vi "createXMLNode.vi"(8 "error in (no error)":errorcluster, 11 "name":string) -> (0 "error out":errorcluster, 3 "xmlNode out":refnum<class "xmlNode.lvclass">)   [LabVIEW 2011, in "Tools.lvlib" / "xml.lvlib" / "xmlNode.lvclass"]
uses:
  xmlNode.lvclass
  xmlNode.lvclass/xmlNode.ctl
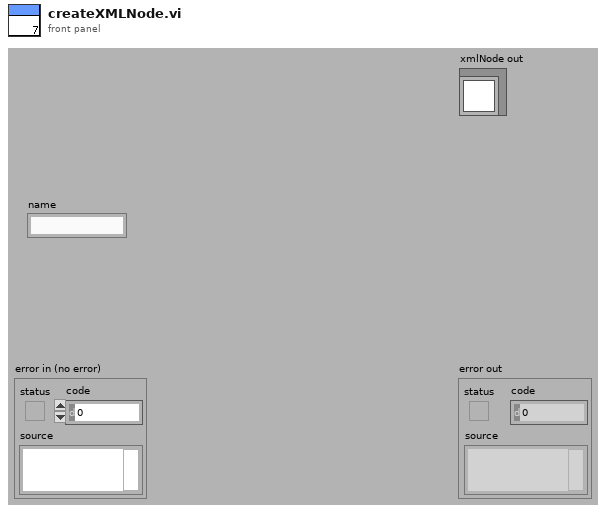
[diagram p1: front panel]
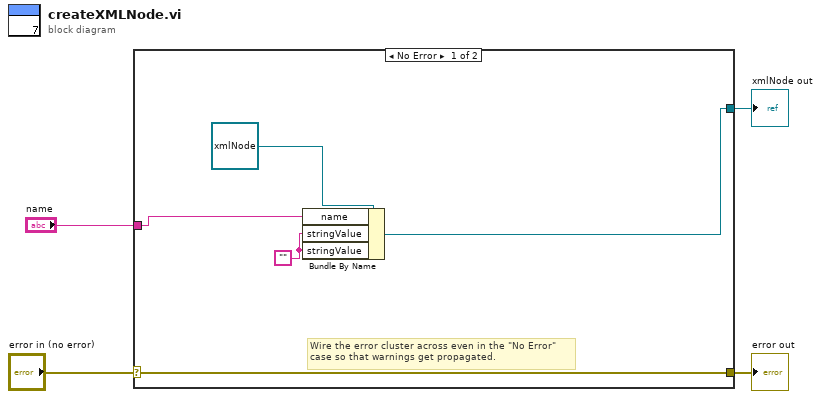
[diagram p0: block diagram]
diagram:
  n1 = case shown="No Error" "error in (no error)" {
    selector: "error in (no error)" -> [w9 w10]
    tunnel: [w9 w10] -> w3
    tunnel: [w6 _] -> w2
    tunnel: "name" -> [w7 _]
    frame No Error {
      w5 = ""
      # "Wire the error cluster across even in the \"No Error\"\ncase so that warnings get propagated."
      n2 = Bundle By Name(cluster=refnum<class "xmlNode.lvclass"> refnum ("Tools.lvlib:xmlNode.lvclass"), "name"=w7, "stringValue"=w5, "stringValue"=w5) -> (w6:refnum<class "xmlNode.lvclass">)
    }
    frame Error {
    }
  }
  "error out" <- w3
  "xmlNode out" <- w2
